vi "Get SMO Vendor.vi"(8 "error in (no error)":errorcluster, 11 "Instrument.Transport in":refnum<class "Inst.Transport.lvclass">) -> (0 "error out":errorcluster, 2 "SMO Vendor":string, 3 "Instrument.Transport out":refnum<class "Inst.Transport.lvclass">)   [LabVIEW 2019, in "Inst.Transport.lvclass"]
doc: "Override this VI to return the vendor or manufacturer of your Instrument"
uses:
  Inst.Transport.lvclass
  <userlib>/LevyLab/Instrument Framework/Instrument Types/SCPI/Instrument.SCPI.lvclass
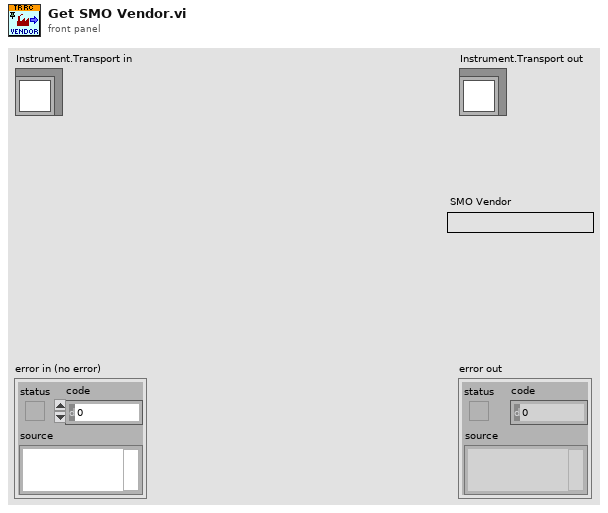
[diagram p1: front panel]
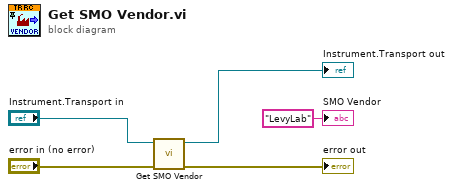
[diagram p0: block diagram]
diagram:
  n1 = call-parent "Get SMO Vendor.vi"("error in (no error)"="error in (no error)", "Instrument in"="Instrument.Transport in") -> ("error out"=→"error out":errorcluster, "Instrument out"=→"Instrument.Transport out":refnum<class "Inst.Transport.lvclass">)  [unwired: 7 in, 1 out]
  "SMO Vendor" <- "LevyLab" ("SMO Vendor")
